vi "movtreeitems.vi"(2 "error out 2":errorcluster, 3 "Array":T1(array[cluster]), 4 "String":string, 5 "Tree 2":refnum<vi>) -> (0 "error out":errorcluster, 1 "Tree":refnum<vi>)   [LabVIEW 2010]
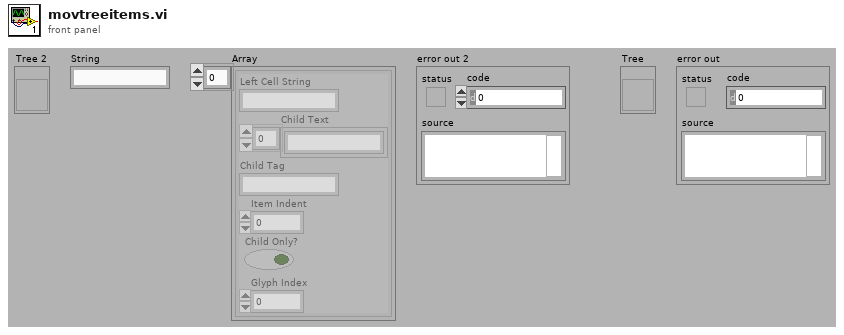
[diagram p1: front panel]
types:
  T1 = cluster{"Left Cell String":string, "Child Text":string[], "Child Tag":string, "Item Indent":i32, "Child Only?":bool, "Glyph Index":i32}[]
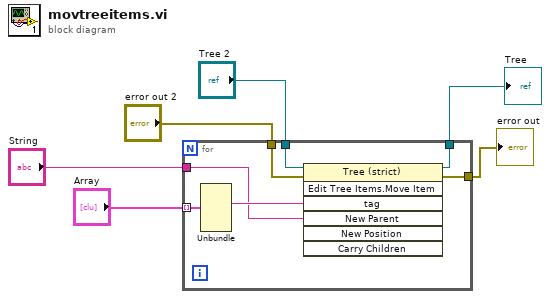
[diagram p0: block diagram]
diagram:
  n1 = for {
    tunnel: "Tree 2" -> [w13]
    tunnel: "error out 2" -> [w12]
    tunnel: [w11] -> w3
    tunnel: [w10] -> w4
    tunnel: "Array" -> [w9] mode=indexing
    tunnel: "String" -> [w7]
    n2 = Unbundle(w9) -> ("Child Tag"=w8:string)  [unwired: 5 out]
    n3 = invoke on="Invoke Node" class="Tree (strict)" method="Edit Tree Items.Move Item"(reference=w13, error in=w12, "tag"=w8, "New Parent"=w7) -> (reference out=w11:refnum<vi>, error out=w10:errorcluster)  [unwired: 3 in, 5 out]
  }
  "error out" <- w4
  "Tree" <- w3
